vi "blokada wysylania jazda.vi"(6 "Y axis":i32, 9 "X axis":i32, 11 "Boolean in":refnum<vi>) -> (1 "zak2":bool, 2 "blokada jazdy":bool, 4 "zak1":bool)   [LabVIEW 2014]
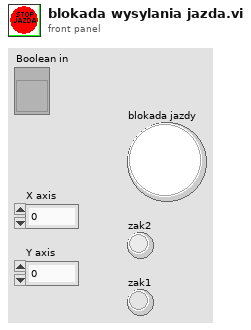
[diagram p1: front panel]
types:
  T1 = enum16{"Rising Edge", "Falling Edge", "Any Edge"}
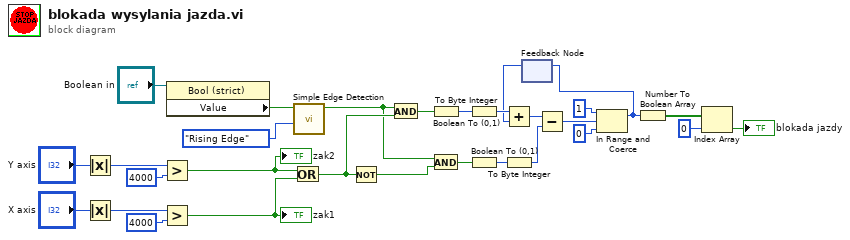
[diagram p0: block diagram]
diagram:
  n1 = Absolute Value(x="Y axis") -> (abs(x)=w20:i32)
  n2 = Absolute Value(x="X axis") -> (abs(x)=w23:i32)
  n3 = Greater?(x=w20, y=4000) -> (0:w28:bool)
  "zak2" <- w28
  n4 = Greater?(x=w23, y=4000) -> (0:w29:bool)
  "zak1" <- w29
  n5 = property class="Bool (strict)"(reference="Boolean in") -> ("Value"=w13:bool)  [unwired: 1 in, 2 out]
  n6 = Or(x=w28, y=w29) -> (x .or. y?=w27:bool)
  n7 = call "Simple Edge Detection.vi"("Mode"=T1."Rising Edge", "clk_in"=w13) -> ("edge?"=w19:bool)  [unwired: 9 in]
  n8 = Not(x=w27) -> (.not. x?=w26:bool)
  n9 = And(x=w19, y=w27) -> (x .and. y?=w17:bool)
  n10 = Boolean To (0,1)(Boolean=w17) -> (0, 1=w6:i16)
  n11 = And(x=w19, y=w26) -> (x .and. y?=w18:bool)
  n12 = To Byte Integer(number=w6) -> (8bit integer=w5:i8)
  n13 = Boolean To (0,1)(Boolean=w18) -> (0, 1=w4:i16)
  n14 = To Byte Integer(number=w4) -> (8bit integer=w3:i8)
  n15 = feedback #1() -> (w1:i8)  [unwired: 1 in]
  n16 = Add(x=w5, y=w1) -> (x+y=w16:i8)
  n17 = Subtract(x=w16, y=w3) -> (x-y=w15:i8)
  n18 = In Range and Coerce(upper limit=i8 1 ("lower limit"), x=w15, lower limit=i8 0) -> (coerced(x)=w2:i8)  [unwired: 1 out]
  n19 = feedback-in #1(w2) -> ()
  n20 = Number To Boolean Array(number=w2) -> (Boolean array=w9:bool[])
  n21 = Index Array(array=w9, index=0) -> (element=→"blokada jazdy":bool)
